vi "Read Destroy.vi"(11 "Base Actor in":refnum<class "Base Actor.lvclass">) -> (2 "Destroy":bool)   [LabVIEW 2020, in "jettl.lvlib" / "Actor.lvlib" / "Base Actor.lvclass"]
uses:
  Base Actor.lvclass
  Base Actor.lvclass/Base Actor.ctl
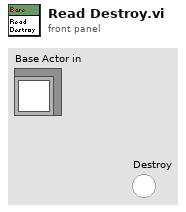
[diagram p1: front panel]
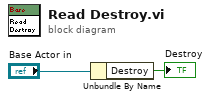
[diagram p0: block diagram]
diagram:
  n1 = Unbundle By Name("Base Actor in") -> ("Destroy"=→"Destroy":bool)
